vi "myRIO v1.0 Configure IO.vi"(7 "Value":bool, 8 "error in (no error)":errorcluster, 10 "Bitmask Array":bool[][](array[boolean]), 11 "myRIO FPGA Ref In":T1) -> (0 "error out":errorcluster)   [LabVIEW 2021]
uses:
  <vilib>/myRIO/Common/Instrument Driver Framework/Utilities/typedefs/Generic FPGA Reference.ctl
  <vilib>/myRIO/Common/Instrument Driver Framework/myRIO v1.0/Resource Manager/typedefs/IO Config FPGA Reference.ctl
  <vilib>/myRIO/Common/Instrument Driver Framework/myRIO v1.0/Resource Manager/typedefs/myRIO v1.0 Connector List.ctl
  <vilib>/Utility/error.llb/Error Cluster From Error Code.vi
  <vilib>/rvi/errors/niLvFpgaAdjustHostInterfaceError.vi
  <vilib>/rvi/interface/nirviReadWriteControl/nirviReadWriteControl.xnode
  <vilib>/rvi/interface/Simulation/niFpgaSimulationCallBeginRW.vi
  NiFpgaLv.dll
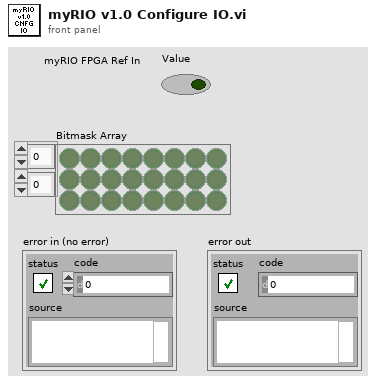
[diagram p1: front panel]
types:
  T1 = typedef "Generic FPGA Reference.ctl" = refnum<k20>
  T2 = typedef "IO Config FPGA Reference.ctl" = refnum<k20>
  T3 = typedef "myRIO v1.0 Connector List.ctl" = enum32{"None", "ConnectorA", "ConnectorB", "ConnectorC"}
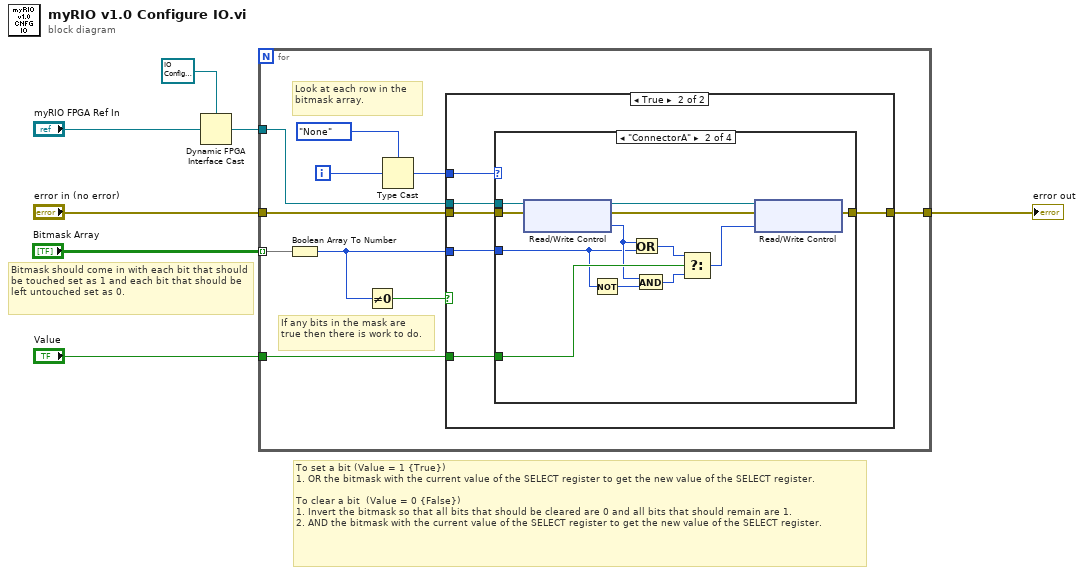
[diagram p0: block diagram]
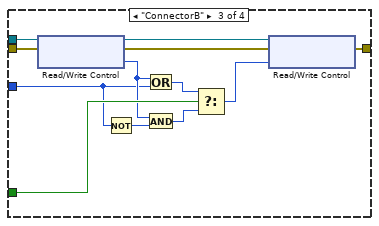
[diagram p4: hidden frame]
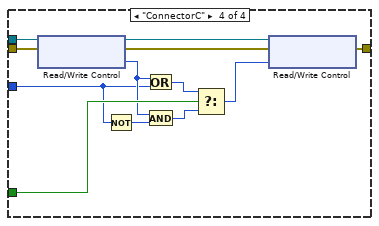
[diagram p5: hidden frame]
diagram:
  # "To set a bit (Value = 1 {True}) \n1. OR the bitmask with the current value of the SELECT register to get the new value of the SELECT register.\n\nTo clear a bit  (Value = 0 {False})\n1. Invert the bitmask so that all bits that should be cleared are 0 and all bits that should remain are 1.\n2. AND the bitmask with the current value of the SELECT register to get the new value of the SELECT register."
  # "Bitmask should come in with each bit that should be touched set as 1 and each bit that should be left untouched set as 0."
  n1 = Dynamic FPGA Interface Cast(Session In=T2 refnum ("FPGA Interface"), Type="myRIO FPGA Ref In") -> (Session Out=w3:T2)
  n2 = for {
    tunnel: w3 -> [w17]
    tunnel: "error in (no error)" -> [w16]
    tunnel: [w15] -> w6
    tunnel: "Bitmask Array" -> [w10] mode=indexing
    tunnel: "Value" -> [w11]
    i -> [w14]
    # "If any bits in the mask are\ntrue then there is work to do."
    # "Look at each row in the bitmask array."
    n3 = Boolean Array To Number(Boolean array=w10) -> (number=w9:u8)
    n4 = Not Equal To 0?(x=w9) -> (x != 0?=w8:bool)
    n5 = Type Cast(type=myRIO_v1.0_Connector_List."None" ("Connector List"), x=w14) -> (*(type *) &x=w13:T3)
    n6 = case shown="True" w8 {
      tunnel: w17 -> [_ w24]
      tunnel: w16 -> [w18 w23]
      tunnel: [w18 w22] -> w15
      tunnel: w13 -> [_ w21]
      tunnel: w9 -> [_ w20]
      tunnel: w11 -> [_ w19]
      frame False {
        # "There are no bits to change for this connector."
      }
      frame True {
        n7 = case shown="\"ConnectorA\"" w21 {
          tunnel: w24 -> [_ w37 w49 w61]
          tunnel: w23 -> [w25 w36 w48 w60]
          tunnel: [w25 w33 w45 w57] -> w22
          tunnel: w20 -> [_ w29 w41 w53]
          tunnel: w19 -> [_ w32 w44 w56]
          frame "None" {
            # "Do Nothing"
          }
          frame "ConnectorA" {
            n8 = xnode "Read/Write Control"("FPGA VI Reference In"=w37, "error in"=w36) -> ("FPGA VI Reference Out"=w34:T2, "error out"=w35:errorcluster, "SYS.SELECTA"=w30:u8)
            n9 = Not(x=w29) -> (.not. x?=w31:u8)
            n10 = Or(x=w30, y=w29) -> (x .or. y?=w27:u8)
            n11 = And(x=w30, y=w31) -> (x .and. y?=w26:u8)
            n12 = Select(t=w27, s=w32, f=w26) -> (s? t:f=w28:u8)
            n13 = xnode "Read/Write Control"("FPGA VI Reference In"=w34, "error in"=w35, "SYS.SELECTA"=w28) -> ("error out"=w33:errorcluster)  [unwired: 1 out]
          }
          frame "ConnectorB" {
            n14 = xnode "Read/Write Control"("FPGA VI Reference In"=w49, "error in"=w48) -> ("FPGA VI Reference Out"=w46:T2, "error out"=w47:errorcluster, "SYS.SELECTB"=w42:u8)
            n15 = Not(x=w41) -> (.not. x?=w43:u8)
            n16 = Or(x=w42, y=w41) -> (x .or. y?=w39:u8)
            n17 = And(x=w42, y=w43) -> (x .and. y?=w38:u8)
            n18 = Select(t=w39, s=w44, f=w38) -> (s? t:f=w40:u8)
            n19 = xnode "Read/Write Control"("FPGA VI Reference In"=w46, "error in"=w47, "SYS.SELECTB"=w40) -> ("error out"=w45:errorcluster)  [unwired: 1 out]
          }
          frame "ConnectorC" {
            n20 = xnode "Read/Write Control"("FPGA VI Reference In"=w61, "error in"=w60) -> ("FPGA VI Reference Out"=w58:T2, "error out"=w59:errorcluster, "SYS.SELECTC"=w54:u8)
            n21 = Not(x=w53) -> (.not. x?=w55:u8)
            n22 = Or(x=w54, y=w53) -> (x .or. y?=w50:u8)
            n23 = And(x=w54, y=w55) -> (x .and. y?=w51:u8)
            n24 = Select(t=w50, s=w56, f=w51) -> (s? t:f=w52:u8)
            n25 = xnode "Read/Write Control"("FPGA VI Reference In"=w58, "error in"=w59, "SYS.SELECTC"=w52) -> ("error out"=w57:errorcluster)  [unwired: 1 out]
          }
        }
      }
    }
  }
  "error out" <- w6
